vi "Write DAQ daemon.vi"(10 "DAQ daemon":refnum<class "Message Enqueuer.lvclass">, 11 "Controller in":refnum<class "Controller.lvclass">) -> (3 "Controller out":refnum<class "Controller.lvclass">)   [LabVIEW 2011, in "Controller.lvclass"]
uses:
  Controller.lvclass
  <userlib>/_Frameworks/ActorFramework/Message Enqueuer/Message Enqueuer.lvclass
  Controller.lvclass/Controller.ctl
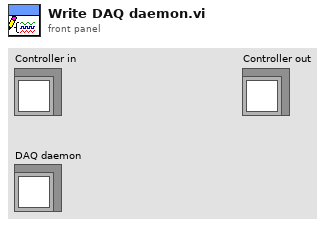
[diagram p1: front panel]
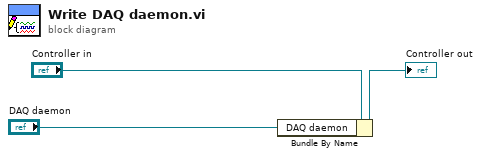
[diagram p0: block diagram]
diagram:
  n1 = Bundle By Name(cluster="Controller in", "DAQ daemon"="DAQ daemon") -> (→"Controller out":refnum<class "Controller.lvclass">)
